vi "Test_sqlite3TableMetadata_ListsTableMetaData.vi"(8 "error in (no error)":errorcluster, 11 "TestCase in":refnum<class "Test sqlite3.lvclass">) -> (0 "error out":errorcluster, 3 "TestCase out":refnum<class "Test sqlite3.lvclass">)   [LabVIEW 2020, in "Test sqlite3.lvclass"]
uses:
  Test sqlite3.lvclass
  Test sqlite3.lvclass/Test sqlite3.ctl
  externals/sqlite3/Source/sqlite3.lvclass
  <vilib>/addons/_JKI Toolkits/VI Tester/TestCase.llb/TestCase.lvclass
  C:/Program Files/National Instruments/LabVIEW 2020/vi.lib/addons/_JKI Toolkits/VI Tester/TestCase.llb/TestCase.lvclass
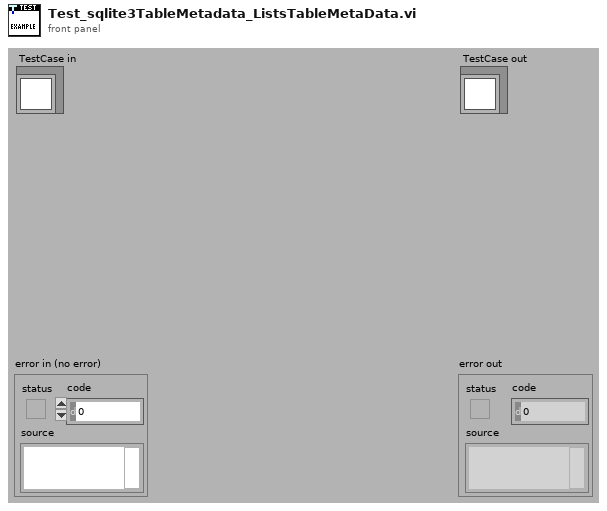
[diagram p1: front panel]
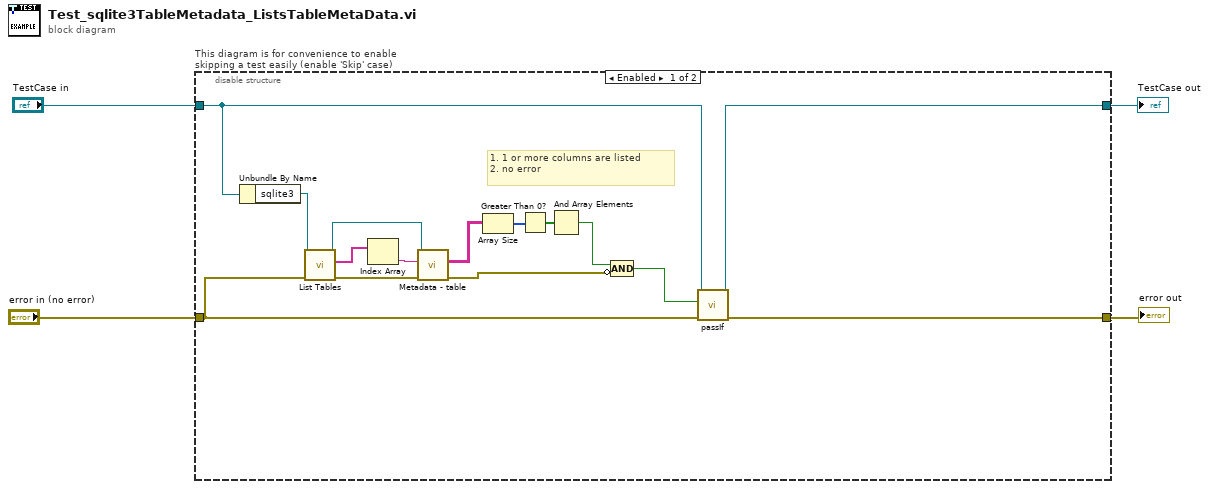
[diagram p0: block diagram]
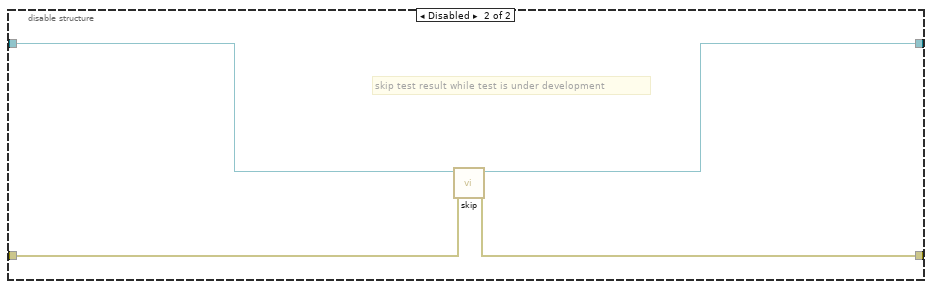
[diagram p2: hidden frame]
diagram:
  n1 = disable-structure "This diagram is for convenience to enable skipping a test easily (enable 'Skip' case)" shown="Enabled" {
    disable-tunnel: "TestCase in" -> [w17 w23]
    disable-tunnel: [w19 w21] -> w1
    disable-tunnel: [w18 w22] -> w3
    disable-tunnel: "error in (no error)" -> [w15 w20]
    frame Enabled {
      # "1. 1 or more columns are listed\n2. no error"
      n2 = Unbundle By Name(w17) -> ("sqlite3"=w16:refnum<class "sqlite3.lvclass">)
      n3 = call-dynamic "List Tables.vi"("error in (no error)"=w15, "sqlite in"=w16) -> ("error out"=w11:errorcluster, "Tables out"=w8:string[], "sqlite out"=w9:refnum<class "sqlite3.lvclass">)  [unwired: 7 in]
      n4 = Index Array(array=w8) -> (element=w7:string)  [unwired: 1 in]
      n5 = call-dynamic "Metadata - table.vi"("error in (no error)"=w11, "Table in"=w7, "sqlite in"=w9) -> ("error out"=w10:errorcluster, "PRAGMA table info"=w6:string[][])  [unwired: 6 in, 1 out]
      n6 = Array Size(array=w6) -> (size(s)=w14:i32[])
      n7 = Greater Than 0?(x=w14) -> (x > 0?=w13:bool[])
      n8 = And Array Elements(Boolean array=w13) -> (logical AND=w5:bool)
      n9 = Compound Arithmetic op=AND(w5, invert w10) -> (w12:bool)
      n10 = call-dynamic "passIf.vi"("error in (no error)"=w15, "pass"=w12, "TestCase in"=w17) -> ("error out"=w18:errorcluster, "TestCase out"=w19:refnum<class "Test sqlite3.lvclass">)  [unwired: 7 in]
    }
    frame Disabled {
      # "skip test result while test is under development"
      n11 = call <vilib>:"skip.vi"("error in (no error)"=w20, "TestCase in"=w23) -> ("error out"=w22:errorcluster, "TestCase out"=w21:refnum<class "Test sqlite3.lvclass">)  [unwired: 8 in]
    }
  }
  "error out" <- w3
  "TestCase out" <- w1
